vi "Read Data Bits.vi"(8 "error in (no error)":errorcluster, 11 "Serial Data Unit in":refnum<class "Serial Data Unit.lvclass">) -> (0 "error out":errorcluster, 2 "data bits":u16=8, 3 "Serial Data Unit out":refnum<class "Serial Data Unit.lvclass">)   [LabVIEW 2012, in "Serial Data Unit.lvclass"]
doc: "Acts as a constant, and provides a way for the serial slave to properly configure the serial interface."
uses:
  Serial Data Unit.lvclass
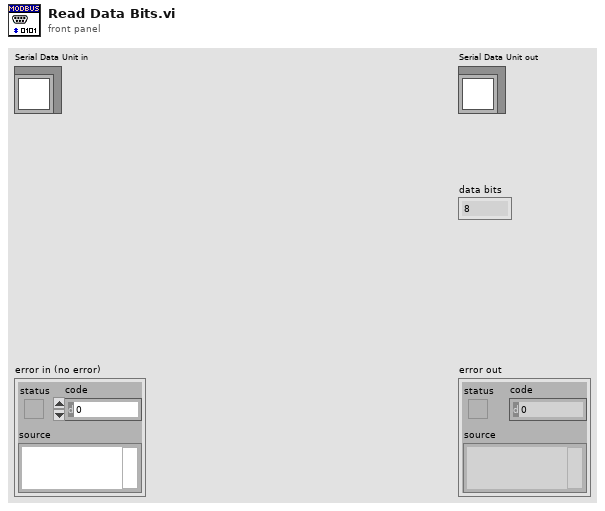
[diagram p1: front panel]
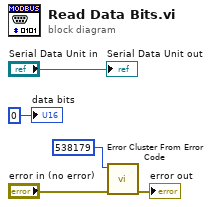
[diagram p0: block diagram]
diagram:
  n1 = call <vilib>:"Error Cluster From Error Code.vi"("error in (no error)"="error in (no error)", "error code (0)"=538179) -> ("error out"=→"error out":errorcluster)  [unwired: 7 in]
  "Serial Data Unit out" <- "Serial Data Unit in"
  "data bits" <- u16 0 ("data bits")
